vi "InstrumentsOrder.vi"(0 "VISA资源名称":refnum<visa-resource-name>, 2 "通道选择 2":u16(ring) items=["CH1", "CH2", "CH3", "CH4"], 5 "错误输入（无错误）":errorcluster) -> (10 "PERIOD":dbl, 11 "FREQ":dbl, 12 "PK2PK":dbl, 14 "VISA资源名称输出":refnum<visa-resource-name>, 15 "Max":dbl, 16 "AMP":dbl, 17 "RMS":dbl, 18 "MIN":dbl, 19 "错误输出":errorcluster)   [LabVIEW 2014]
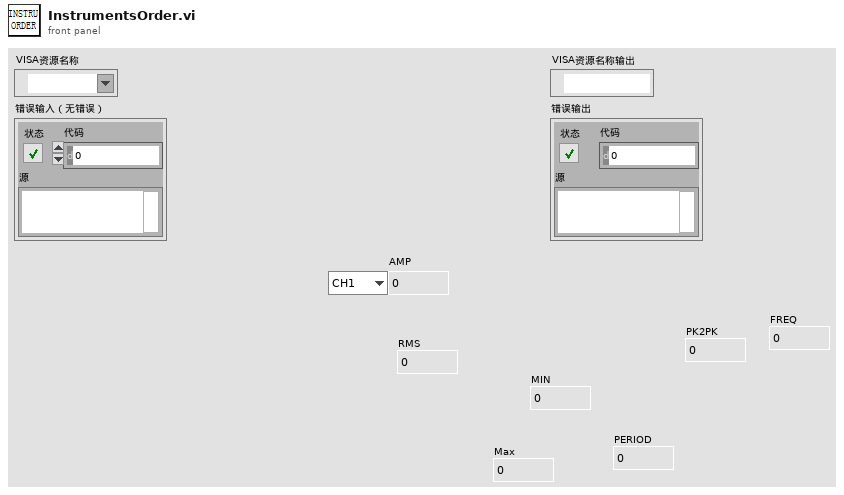
[diagram p1: front panel]
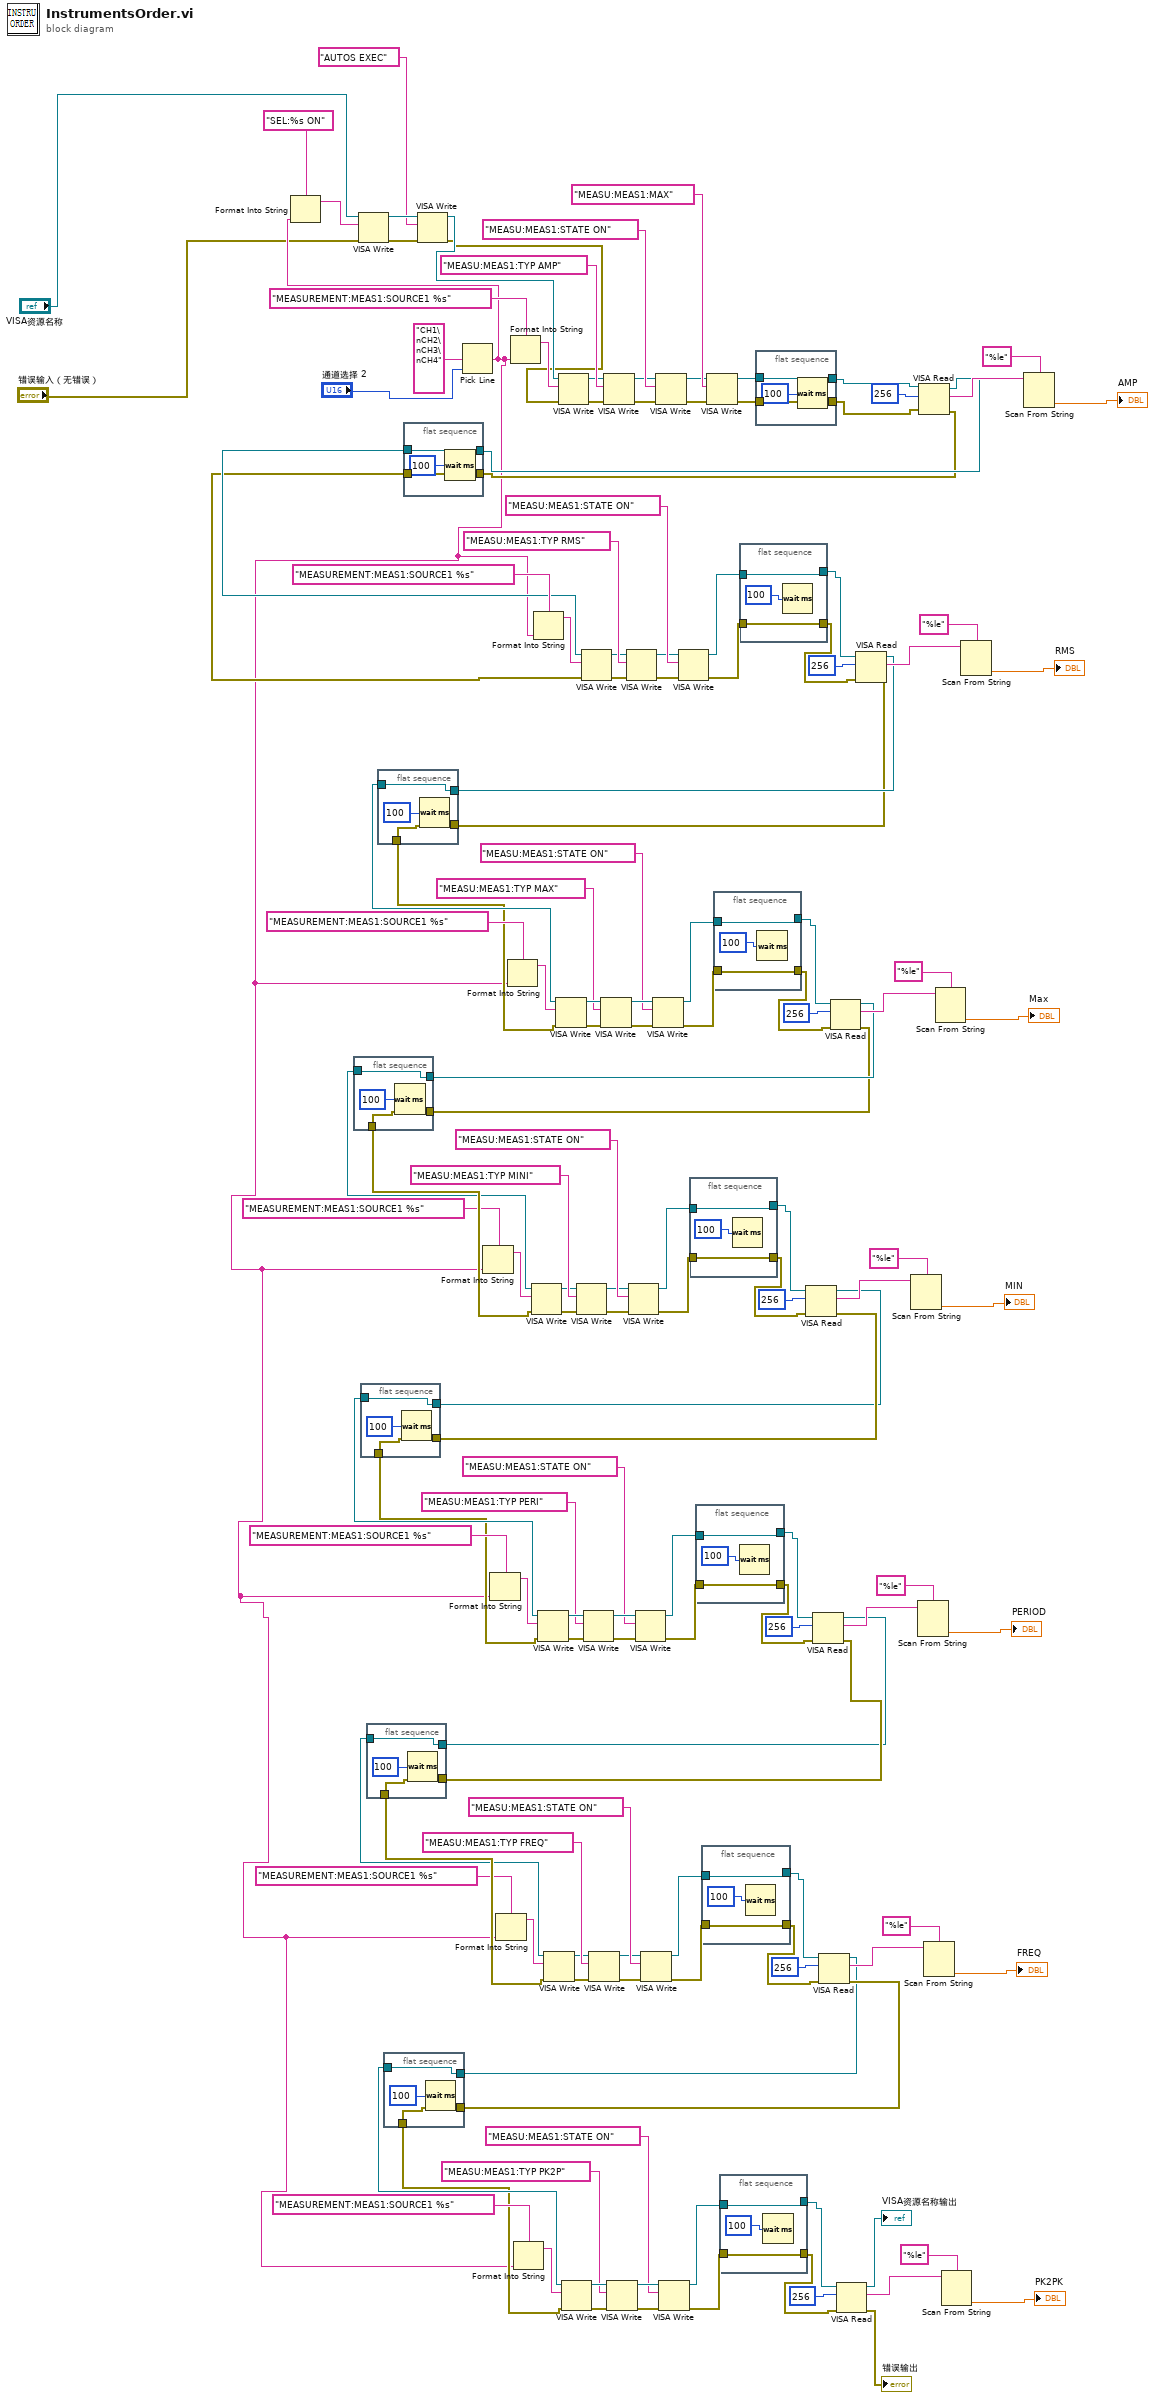
[diagram p0: block diagram]
diagram:
  n1 = flat-sequence {
    tunnel: w74 -> [w155]
    tunnel: [w155] -> w91
    tunnel: w73 -> [w154]
    tunnel: [w154] -> w92
    frame #0 {
      n2 = Wait (ms)(milliseconds to wait=u32 100 ("等待时间（毫秒）")) -> ()  [unwired: 1 out]
    }
  }
  n3 = flat-sequence {
    tunnel: w53 -> [w158]
    tunnel: [w158] -> w56
    tunnel: w54 -> [w157]
    tunnel: [w157] -> w55
    frame #0 {
      n4 = Wait (ms)(milliseconds to wait=u32 100 ("等待时间（毫秒）")) -> ()  [unwired: 1 out]
    }
  }
  n5 = flat-sequence {
    tunnel: w33 -> [w161]
    tunnel: [w161] -> w51
    tunnel: w34 -> [w160]
    tunnel: [w160] -> w52
    frame #0 {
      n6 = Wait (ms)(milliseconds to wait=u32 100 ("等待时间（毫秒）")) -> ()  [unwired: 1 out]
    }
  }
  n7 = flat-sequence {
    tunnel: w96 -> [w164]
    tunnel: [w164] -> w95
    tunnel: w94 -> [w163]
    tunnel: [w163] -> w93
    frame #0 {
      n8 = Wait (ms)(milliseconds to wait=u32 100 ("等待时间（毫秒）")) -> ()  [unwired: 1 out]
    }
  }
  n9 = flat-sequence {
    tunnel: w13 -> [w167]
    tunnel: [w167] -> w16
    tunnel: w14 -> [w166]
    tunnel: [w166] -> w15
    frame #0 {
      n10 = Wait (ms)(milliseconds to wait=u32 100 ("等待时间（毫秒）")) -> ()  [unwired: 1 out]
    }
  }
  n11 = flat-sequence {
    tunnel: w116 -> [w171]
    tunnel: [w171] -> w114
    tunnel: [w170] -> w113
    tunnel: w115 -> [w170]
    frame #0 {
      n12 = Wait (ms)(milliseconds to wait=u32 100 ("等待时间（毫秒）")) -> ()  [unwired: 1 out]
    }
  }
  n13 = Pick Line(multi-line string="CH1\nCH2\nCH3\nCH4" ("多行字符串"), line index="通道选择 2") -> (output string=w5:string)  [unwired: 1 in]
  n14 = Format Into String(format string="SEL:%s ON" ("格式字符串"), w5) -> (resulting string=w7:string)  [unwired: 2 in, 1 out]
  n15 = VISA Write(VISA resource name="VISA资源名称", write buffer=w7, error in (no error)="错误输入（无错误）") -> (VISA resource name out=w9:refnum<visa-resource-name>, error out=w10:errorcluster)  [unwired: 1 out]
  n16 = VISA Write(VISA resource name=w9, write buffer="AUTOS EXEC" ("写入缓冲区"), error in (no error)=w10) -> (VISA resource name out=w2:refnum<visa-resource-name>, error out=w1:errorcluster)  [unwired: 1 out]
  n17 = Format Into String(format string="MEASUREMENT:MEAS1:SOURCE1 %s" ("格式字符串"), w5) -> (resulting string=w81:string)  [unwired: 2 in, 1 out]
  n18 = Format Into String(format string="MEASUREMENT:MEAS1:SOURCE1 %s" ("格式字符串"), w5) -> (resulting string=w66:string)  [unwired: 2 in, 1 out]
  n19 = Format Into String(format string="MEASUREMENT:MEAS1:SOURCE1 %s" ("格式字符串"), w5) -> (resulting string=w41:string)  [unwired: 2 in, 1 out]
  n20 = Format Into String(format string="MEASUREMENT:MEAS1:SOURCE1 %s" ("格式字符串"), w5) -> (resulting string=w106:string)  [unwired: 2 in, 1 out]
  n21 = Format Into String(format string="MEASUREMENT:MEAS1:SOURCE1 %s" ("格式字符串"), w5) -> (resulting string=w146:string)  [unwired: 2 in, 1 out]
  n22 = Format Into String(format string="MEASUREMENT:MEAS1:SOURCE1 %s" ("格式字符串"), w5) -> (resulting string=w26:string)  [unwired: 2 in, 1 out]
  n23 = VISA Write(VISA resource name=w91, write buffer=w81, error in (no error)=w92) -> (VISA resource name out=w79:refnum<visa-resource-name>, error out=w78:errorcluster)  [unwired: 1 out]
  n24 = Format Into String(format string="MEASUREMENT:MEAS1:SOURCE1 %s" ("格式字符串"), w5) -> (resulting string=w127:string)  [unwired: 2 in, 1 out]
  n25 = VISA Write(VISA resource name=w56, write buffer=w66, error in (no error)=w55) -> (VISA resource name out=w68:refnum<visa-resource-name>, error out=w69:errorcluster)  [unwired: 1 out]
  n26 = VISA Write(VISA resource name=w51, write buffer=w41, error in (no error)=w52) -> (VISA resource name out=w39:refnum<visa-resource-name>, error out=w38:errorcluster)  [unwired: 1 out]
  n27 = VISA Write(VISA resource name=w95, write buffer=w106, error in (no error)=w93) -> (VISA resource name out=w108:refnum<visa-resource-name>, error out=w109:errorcluster)  [unwired: 1 out]
  n28 = VISA Write(VISA resource name=w2, write buffer=w146, error in (no error)=w1) -> (VISA resource name out=w144:refnum<visa-resource-name>, error out=w143:errorcluster)  [unwired: 1 out]
  n29 = VISA Write(VISA resource name=w16, write buffer=w26, error in (no error)=w15) -> (VISA resource name out=w28:refnum<visa-resource-name>, error out=w29:errorcluster)  [unwired: 1 out]
  n30 = VISA Write(VISA resource name=w79, write buffer="MEASU:MEAS1:TYP MINI" ("写入缓冲区"), error in (no error)=w78) -> (VISA resource name out=w76:refnum<visa-resource-name>, error out=w75:errorcluster)  [unwired: 1 out]
  n31 = VISA Write(VISA resource name=w114, write buffer=w127, error in (no error)=w113) -> (VISA resource name out=w125:refnum<visa-resource-name>, error out=w124:errorcluster)  [unwired: 1 out]
  n32 = VISA Write(VISA resource name=w68, write buffer="MEASU:MEAS1:TYP PERI" ("写入缓冲区"), error in (no error)=w69) -> (VISA resource name out=w71:refnum<visa-resource-name>, error out=w72:errorcluster)  [unwired: 1 out]
  n33 = VISA Write(VISA resource name=w39, write buffer="MEASU:MEAS1:TYP FREQ" ("写入缓冲区"), error in (no error)=w38) -> (VISA resource name out=w36:refnum<visa-resource-name>, error out=w35:errorcluster)  [unwired: 1 out]
  n34 = VISA Write(VISA resource name=w108, write buffer="MEASU:MEAS1:TYP MAX" ("写入缓冲区"), error in (no error)=w109) -> (VISA resource name out=w111:refnum<visa-resource-name>, error out=w112:errorcluster)  [unwired: 1 out]
  n35 = VISA Write(VISA resource name=w144, write buffer="MEASU:MEAS1:TYP AMP" ("写入缓冲区"), error in (no error)=w143) -> (VISA resource name out=w141:refnum<visa-resource-name>, error out=w140:errorcluster)  [unwired: 1 out]
  n36 = VISA Write(VISA resource name=w28, write buffer="MEASU:MEAS1:TYP PK2P" ("写入缓冲区"), error in (no error)=w29) -> (VISA resource name out=w31:refnum<visa-resource-name>, error out=w32:errorcluster)  [unwired: 1 out]
  n37 = VISA Write(VISA resource name=w125, write buffer="MEASU:MEAS1:TYP RMS" ("写入缓冲区"), error in (no error)=w124) -> (VISA resource name out=w122:refnum<visa-resource-name>, error out=w121:errorcluster)  [unwired: 1 out]
  n38 = VISA Write(VISA resource name=w76, write buffer="MEASU:MEAS1:STATE ON" ("写入缓冲区"), error in (no error)=w75) -> (VISA resource name out=w87:refnum<visa-resource-name>, error out=w89:errorcluster)  [unwired: 1 out]
  n39 = VISA Write(VISA resource name=w71, write buffer="MEASU:MEAS1:STATE ON" ("写入缓冲区"), error in (no error)=w72) -> (VISA resource name out=w60:refnum<visa-resource-name>, error out=w58:errorcluster)  [unwired: 1 out]
  n40 = VISA Write(VISA resource name=w36, write buffer="MEASU:MEAS1:STATE ON" ("写入缓冲区"), error in (no error)=w35) -> (VISA resource name out=w47:refnum<visa-resource-name>, error out=w49:errorcluster)  [unwired: 1 out]
  n41 = VISA Write(VISA resource name=w111, write buffer="MEASU:MEAS1:STATE ON" ("写入缓冲区"), error in (no error)=w112) -> (VISA resource name out=w100:refnum<visa-resource-name>, error out=w98:errorcluster)  [unwired: 1 out]
  n42 = VISA Write(VISA resource name=w141, write buffer="MEASU:MEAS1:STATE ON" ("写入缓冲区"), error in (no error)=w140) -> (VISA resource name out=w138:refnum<visa-resource-name>, error out=w137:errorcluster)  [unwired: 1 out]
  n43 = VISA Write(VISA resource name=w31, write buffer="MEASU:MEAS1:STATE ON" ("写入缓冲区"), error in (no error)=w32) -> (VISA resource name out=w20:refnum<visa-resource-name>, error out=w18:errorcluster)  [unwired: 1 out]
  n44 = VISA Write(VISA resource name=w122, write buffer="MEASU:MEAS1:STATE ON" ("写入缓冲区"), error in (no error)=w121) -> (VISA resource name out=w133:refnum<visa-resource-name>, error out=w135:errorcluster)  [unwired: 1 out]
  n45 = flat-sequence {
    tunnel: w87 -> [w174]
    tunnel: [w174] -> w88
    tunnel: w89 -> [w173]
    tunnel: [w173] -> w90
    frame #0 {
      n46 = Wait (ms)(milliseconds to wait=u32 100 ("等待时间（毫秒）")) -> ()  [unwired: 1 out]
    }
  }
  n47 = flat-sequence {
    tunnel: w60 -> [w177]
    tunnel: [w177] -> w59
    tunnel: w58 -> [w176]
    tunnel: [w176] -> w57
    frame #0 {
      n48 = Wait (ms)(milliseconds to wait=u32 100 ("等待时间（毫秒）")) -> ()  [unwired: 1 out]
    }
  }
  n49 = flat-sequence {
    tunnel: w47 -> [w180]
    tunnel: [w180] -> w48
    tunnel: w49 -> [w179]
    tunnel: [w179] -> w50
    frame #0 {
      n50 = Wait (ms)(milliseconds to wait=u32 100 ("等待时间（毫秒）")) -> ()  [unwired: 1 out]
    }
  }
  n51 = VISA Write(VISA resource name=w138, write buffer="MEASU:MEAS1:MAX" ("写入缓冲区"), error in (no error)=w137) -> (VISA resource name out=w120:refnum<visa-resource-name>, error out=w118:errorcluster)  [unwired: 1 out]
  n52 = flat-sequence {
    tunnel: w100 -> [w183]
    tunnel: [w183] -> w99
    tunnel: w98 -> [w182]
    tunnel: [w182] -> w97
    frame #0 {
      n53 = Wait (ms)(milliseconds to wait=u32 100 ("等待时间（毫秒）")) -> ()  [unwired: 1 out]
    }
  }
  n54 = flat-sequence {
    tunnel: w20 -> [w186]
    tunnel: [w186] -> w19
    tunnel: w18 -> [w185]
    tunnel: [w185] -> w17
    frame #0 {
      n55 = Wait (ms)(milliseconds to wait=u32 100 ("等待时间（毫秒）")) -> ()  [unwired: 1 out]
    }
  }
  n56 = flat-sequence {
    tunnel: w133 -> [w189]
    tunnel: [w189] -> w134
    tunnel: w135 -> [w188]
    tunnel: [w188] -> w136
    frame #0 {
      n57 = Wait (ms)(milliseconds to wait=u32 100 ("等待时间（毫秒）")) -> ()  [unwired: 1 out]
    }
  }
  n58 = flat-sequence {
    tunnel: [w192] -> w119
    tunnel: w120 -> [w192]
    tunnel: w118 -> [w191]
    tunnel: [w191] -> w117
    frame #0 {
      n59 = Wait (ms)(milliseconds to wait=u32 100 ("等待时间（毫秒）")) -> ()  [unwired: 1 out]
    }
  }
  n60 = VISA Read(VISA resource name=w88, byte count=u32 256 ("字节总数"), error in (no error)=w90) -> (VISA resource name out=w53:refnum<visa-resource-name>, read buffer=w85:string, error out=w54:errorcluster)  [unwired: 1 out]
  n61 = VISA Read(VISA resource name=w59, byte count=u32 256 ("字节总数"), error in (no error)=w57) -> (VISA resource name out=w33:refnum<visa-resource-name>, read buffer=w62:string, error out=w34:errorcluster)  [unwired: 1 out]
  n62 = VISA Read(VISA resource name=w48, byte count=u32 256 ("字节总数"), error in (no error)=w50) -> (VISA resource name out=w13:refnum<visa-resource-name>, read buffer=w45:string, error out=w14:errorcluster)  [unwired: 1 out]
  n63 = VISA Read(VISA resource name=w99, byte count=u32 256 ("字节总数"), error in (no error)=w97) -> (VISA resource name out=w74:refnum<visa-resource-name>, read buffer=w102:string, error out=w73:errorcluster)  [unwired: 1 out]
  n64 = VISA Read(VISA resource name=w19, byte count=u32 256 ("字节总数"), error in (no error)=w17) -> (VISA resource name out=→"VISA资源名称输出":refnum<visa-resource-name>, read buffer=w22:string, error out=→"错误输出":errorcluster)  [unwired: 1 out]
  n65 = VISA Read(VISA resource name=w134, byte count=u32 256 ("字节总数"), error in (no error)=w136) -> (VISA resource name out=w96:refnum<visa-resource-name>, read buffer=w131:string, error out=w94:errorcluster)  [unwired: 1 out]
  n66 = Scan From String(format string="%le" ("格式字符串"), input string=w85) -> (output 1=→"MIN":dbl)  [unwired: 3 in, 3 out]
  n67 = Scan From String(format string="%le" ("格式字符串"), input string=w62) -> (output 1=→"PERIOD":dbl)  [unwired: 3 in, 3 out]
  n68 = VISA Read(VISA resource name=w119, byte count=u32 256 ("字节总数"), error in (no error)=w117) -> (VISA resource name out=w116:refnum<visa-resource-name>, read buffer=w152:string, error out=w115:errorcluster)  [unwired: 1 out]
  n69 = Scan From String(format string="%le" ("格式字符串"), input string=w45) -> (output 1=→"FREQ":dbl)  [unwired: 3 in, 3 out]
  n70 = Scan From String(format string="%le" ("格式字符串"), input string=w102) -> (output 1=→"Max":dbl)  [unwired: 3 in, 3 out]
  n71 = Scan From String(format string="%le" ("格式字符串"), input string=w22) -> (output 1=→"PK2PK":dbl)  [unwired: 3 in, 3 out]
  n72 = Scan From String(format string="%le" ("格式字符串"), input string=w131) -> (output 1=→"RMS":dbl)  [unwired: 3 in, 3 out]
  n73 = Scan From String(format string="%le" ("格式字符串"), input string=w152) -> (output 1=→"AMP":dbl)  [unwired: 3 in, 3 out]
